vi "Set Camera Configuration.vi"(8 "error in (no error)":errorcluster, 11 "CCDCamera in":refnum<class "CCDCamera.lvclass">) -> (0 "error out":errorcluster, 3 "CCDCamera out":refnum<class "CCDCamera.lvclass">)   [LabVIEW 2018, in "CCDCamera.lvclass"]
uses:
  CCDCamera.lvclass
  <userlib>/atmcd32d.llb/Shutter_type typedef.ctl
  <userlib>/atmcd32d.llb/ReadMode_mode typedef.ctl
  <userlib>/atmcd32d.llb/AcquisitionMode_mode typedef.ctl
  CCDCamera.lvclass/CCDCamera.ctl
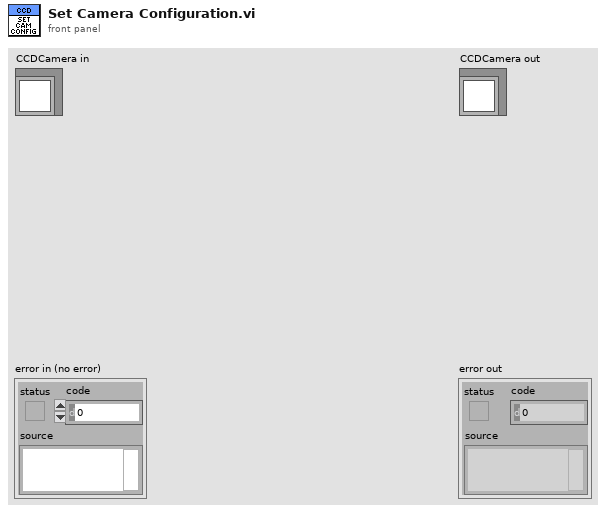
[diagram p1: front panel]
types:
  T1 = typedef "AcquisitionMode_mode typedef.ctl" = enum16{"Reserved (0)", "Single Scan", "Accumulate", "Kinetics", "Fast Kinetics", "Run Till Abort", "Reserved (6)", "Reserved (7)", "Reserved (8)", "Time Delayed Integration"}
  T2 = typedef "ReadMode_mode typedef.ctl" = enum16{"Full Vertical Binning", "Multi-Track", "Random-Track", "Single-Track", "Image"}
  T3 = typedef "Shutter_type typedef.ctl" = enum16{"TTL Low", "TTL High"}
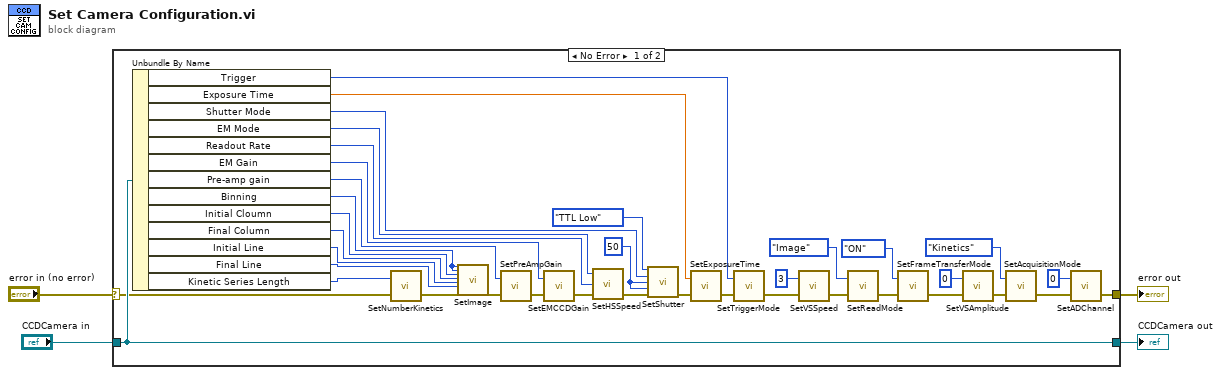
[diagram p0: block diagram]
diagram:
  n1 = case shown="No Error" "error in (no error)" {
    selector: "error in (no error)" -> [w35 w43]
    tunnel: [w14 w43] -> w4
    tunnel: [w36 w42] -> w3
    tunnel: "CCDCamera in" -> [w36 w42]
    frame No Error {
      w21 = 50 ("openingtime")
      n2 = Unbundle By Name(w36) -> ("Trigger"=w5:u16, "Exposure Time"=w11:sgl, "Shutter Mode"=w23:u8, "EM Mode"=w24:u8, "Readout Rate"=w25:u8, "EM Gain"=w26:u16, "Pre-amp gain"=w28:u8, "Binning"=w9:u16, "Initial Cloumn"=w33:u16, "Final Column"=w32:u16, "Initial Line"=w31:u16, "Final Line"=w30:u16, "Kinetic Series Length"=w34:u32)
      n3 = call <userlib>:"SetNumberKinetics.vi"("error in (no error)"=w35, "number"=w34) -> ("error out"=w29:errorcluster)  [unwired: 1 out]
      n4 = call <userlib>:"SetImage.vi"("hbin"=w9, "vbin"=w9, "hstart"=w33, "hend"=w32, "vstart"=w31, "vend"=w30, "error in (no error)"=w29) -> ("error out"=w27:errorcluster)  [unwired: 19 in, 1 out]
      n5 = call <userlib>:"SetPreAmpGain.vi"("error in (no error)"=w27, "index"=w28) -> ("error out"=w37:errorcluster)  [unwired: 1 out]
      n6 = call <userlib>:"SetEMCCDGain.vi"("error in (no error)"=w37, "gain"=w26) -> ("error out"=w38:errorcluster)  [unwired: 1 out]
      n7 = call <userlib>:"SetHSSpeed.vi"("error in (no error)"=w38, "index"=w25, "type"=w24) -> ("error out"=w39:errorcluster)  [unwired: 1 in, 1 out]
      n8 = call <userlib>:"SetShutter.vi"("type"=Shutter_type_typedef."TTL Low", "mode"=w23, "closingtime"=w21, "openingtime"=w21, "error in (no error)"=w39) -> ("error out"=w12:errorcluster)  [unwired: 9 in, 1 out]
      n9 = call <userlib>:"SetExposureTime.vi"("error in (no error)"=w12, "time"=w11) -> ("error out"=w7:errorcluster)  [unwired: 1 out]
      n10 = call <userlib>:"SetTriggerMode.vi"("error in (no error)"=w7, "mode"=w5) -> ("error out"=w6:errorcluster)  [unwired: 1 out]
      n11 = call <userlib>:"SetVSSpeed.vi"("error in (no error)"=w6, "index"=3) -> ("error out"=w40:errorcluster)  [unwired: 1 out]
      n12 = call <userlib>:"SetReadMode.vi"("error in (no error)"=w40, "mode"=ReadMode_mode_typedef."Image") -> ("error out"=w18:errorcluster)  [unwired: 1 out]
      n13 = call <userlib>:"SetFrameTransferMode.vi"("error in (no error)"=w18, "mode"=enum16{"OFF", "ON"}."ON") -> ("error out"=w16:errorcluster)  [unwired: 1 out]
      n14 = call <userlib>:"SetVSAmplitude.vi"("error in (no error)"=w16, "amplitude"=0) -> ("error out"=w8:errorcluster)  [unwired: 1 out]
      n15 = call <userlib>:"SetAcquisitionMode.vi"("error in (no error)"=w8, "mode"=AcquisitionMode_mode_typedef."Kinetics") -> ("error out"=w10:errorcluster)  [unwired: 1 out]
      n16 = call <userlib>:"SetADChannel.vi"("error in (no error)"=w10, "channel"=0) -> ("error out"=w14:errorcluster)  [unwired: 1 out]
    }
    frame Error {
    }
  }
  "error out" <- w4
  "CCDCamera out" <- w3
